vi "Current NED.vi"() -> ()   [LabVIEW 2011]
panel:
  in  "Heading [Deg]":dbl
  in  "Depth [m]":dbl
  in  "East [m]":dbl
  in  "North [m]":dbl
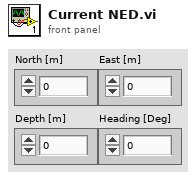
[diagram p1: front panel]
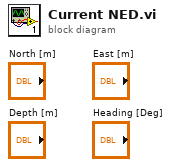
[diagram p0: block diagram]
diagram:
